vi "Trigger.vi"(0 "VISA resource name":refnum<visa-resource-name>, 5 "Command (0: Bus Trigger)":u16(ring) items=["Bus Trigger", "Abort Trigger"], 11 "error in (no error)":errorcluster) -> (4 "VISA resource name out":refnum<visa-resource-name>, 15 "error out":errorcluster)   [LabVIEW 2020, in "Keithley 27XX.lvlib"]
doc: "This VI can either send a Bus Trigger, or Abort a trigger."
uses:
  Keithley 27XX.lvlib
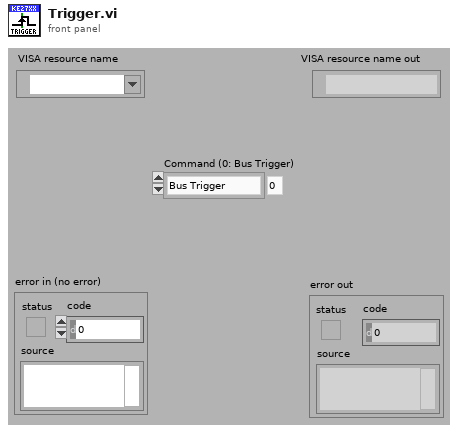
[diagram p1: front panel]
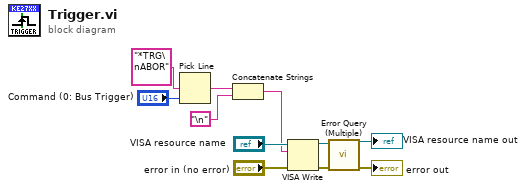
[diagram p0: block diagram]
diagram:
  n1 = Pick Line(multi-line string="*TRG\nABOR", line index="Command (0: Bus Trigger)") -> (output string=w3:string)  [unwired: 1 in]
  n2 = Concatenate Strings(w3, "\n") -> (w2:string)
  n3 = VISA Write(VISA resource name="VISA resource name", write buffer=w2, error in (no error)="error in (no error)") -> (VISA resource name out=w7:refnum<visa-resource-name>, error out=w6:errorcluster)  [unwired: 1 out]
  n4 = call "Error Query (Multiple).vi"("VISA resource name"=w7, "error in (no error)"=w6) -> ("VISA resource name out"=→"VISA resource name out":refnum<visa-resource-name>, "error out"=→"error out":errorcluster)  [unwired: 10 in, 2 out]
